vi "call on write tree.vi"(8 "error in":errorcluster, 11 "root":T1) -> (0 "error out":errorcluster)   [LabVIEW 2023, in "CEF.lvlib" / "CEF_HierarchyRepo.lvclass"]
doc: "Copyright 2017 National Instruments Corporation\n\nLicensed under the Apache License, Version 2.0 (the \"License\"); you may not use this file except in compliance with the License. You may obtain a copy of the License at http://www.apache.org/licenses/LICENSE-2.0\nUnless required by applicable law or agreed to in writing, software distributed under the License is distributed on an \"AS IS\" BASIS, WITHOUT WARRANTIES OR CONDITIONS OF ANY KIND, either express or implied. See the License for the specific language governing permissions and limitations under the License."
uses:
  CEF_HierarchyRepo.lvclass
  Node/NodeRef.ctl
  Node/CEF_Node.lvclass
  Node/CEF_Node.lvclass/CEF_Node.ctl
  Node/ReadChildren.vi
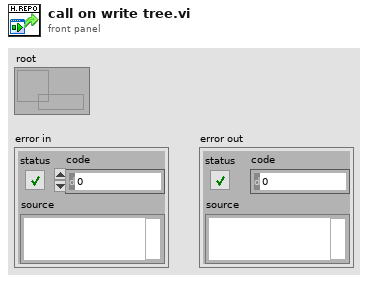
[diagram p1: front panel]
types:
  T1 = typedef "CEF.lvlib/CEF_Node.lvclass/NodeRef.ctl" = refnum<data-value>
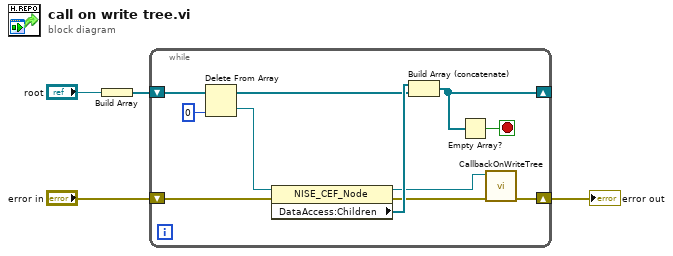
[diagram p0: block diagram]
diagram:
  n1 = Build Array("root") -> (w4:T1[])
  n2 = while {
    shift-right: [w5] -> w2
    shift-left: "error in" -> [w13]
    shift-right: [w9] -> _
    shift-left: w4 -> [w15]
    stop <- w8 stop-if-true
    n3 = Delete From Array(array=w15, index=0) -> (deleted portion=w12:T1, array with subset deleted=w10:T1[])  [unwired: 1 in]
    n4 = property class="NISE_CEF_Node"(reference=w12, error in=w13) -> (reference out=w7:T1, error out=w6:errorcluster, "DataAccess:Children"=w11:T1[])
    n5 = Build Array (concatenate)(w11, w10) -> (w9:T1[])
    n6 = Empty Array?(array=w9) -> (empty?=w8:bool)
    n7 = call "CallbackOnWriteTree.vi"("error in"=w6, "node"=w7) -> ("error out"=w5:errorcluster)  [unwired: 9 in]
  }
  "error out" <- w2
